vi "Logger.vi"(8 "error in":errorcluster, 10 "Path":path=path "C:/Users/ipova/repos/labview/MGI_AFTutorial/Files", 11 "Logger.lvlib:Logger.lvclass 2":refnum<class "Logger.lvclass">) -> (0 "error out":errorcluster, 3 "Logger.lvlib:Logger.lvclass":refnum<class "Logger.lvclass">)   [LabVIEW 2020, in "Logger.lvlib" / "Logger.lvclass"]
uses:
  Logger.lvclass
  Logger.lvclass/Logger.ctl
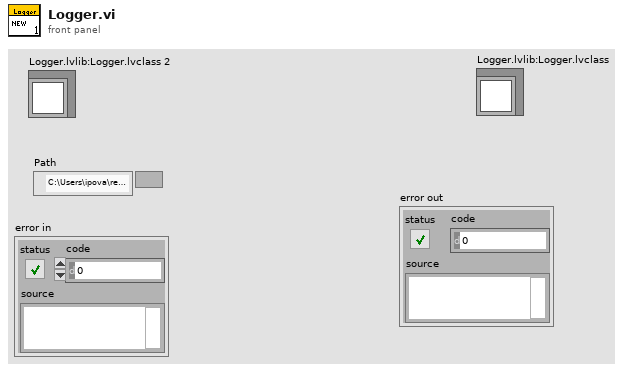
[diagram p1: front panel]
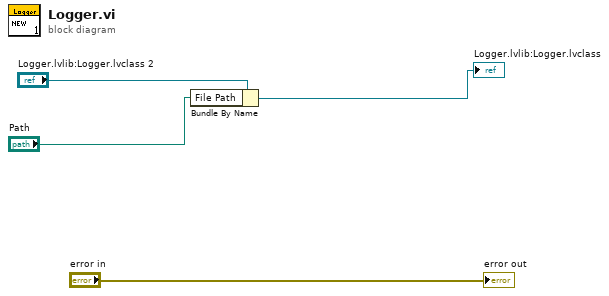
[diagram p0: block diagram]
diagram:
  n1 = Bundle By Name(cluster="Logger.lvlib:Logger.lvclass 2", "File Path"="Path") -> (→"Logger.lvlib:Logger.lvclass":refnum<class "Logger.lvclass">)
  "error out" <- "error in"
